vi "Parse Full Path or Item Name.vi"(11 "Full Path (with $) or Name":string) -> (3 "Relative Path or JSON-format name":string)   [LabVIEW 2017, in "JSONtext.lvlib"]
uses:
  JSONtext.lvlib
  support/quote and escape json string 2.vi
  <vilib>/JDP Science/JDP Science Common Utilities/JDP Utility.lvlib
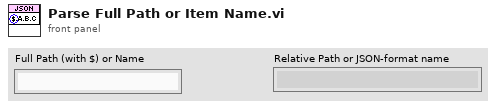
[diagram p1: front panel]
types:
  T1 = typedef "JSONtext.lvlib/Parsing State.ctl" = enum16{"Parser Error", "Object", "Array", "String", "Number/Other", "Leading Whitespace", "Object end", "Array end", "Value end"}
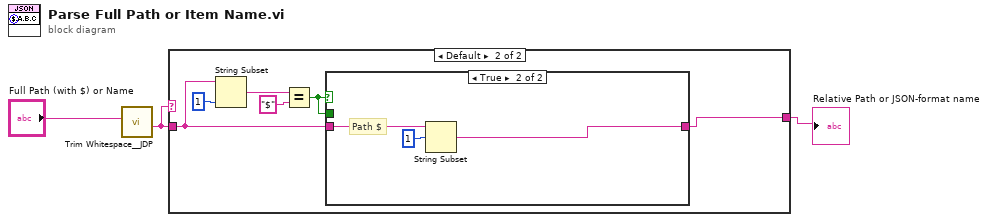
[diagram p0: block diagram]
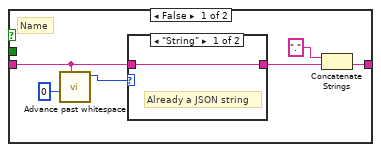
[diagram p3: hidden frame]
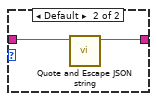
[diagram p4: hidden frame]
diagram:
  n1 = call <vilib>:"Trim Whitespace__JDP.vi"("String in"="Full Path (with $) or Name") -> ("String out"=w2:string)  [unwired: 6 in]
  n2 = case shown="Default" w2 {
    tunnel: w2 -> [_ w5]
    tunnel: [_ w4] -> w1
    frame "" {
    }
    frame Default {
      n3 = String Subset(string=w5, length (rest)=1 ("length (rest)")) -> (substring=w9:string)  [unwired: 1 in]
      n4 = Equal?(x=w9, y="$") -> (x = y?=w6:bool)
      n5 = case shown="True" w6 {
        tunnel: w6 -> [_ _]
        tunnel: w5 -> [w15 w21]
        tunnel: [w10 w19] -> w4
        frame False {
          # "Name"
          n6 = call "Advance past whitespace.vi"("JSON"=w15, "Offset"=0) -> ("Parser State"=w13:T1)  [unwired: 8 in, 1 out]
          n7 = case shown="\"String\"" w13 {
            tunnel: [w16 w18] -> w11
            tunnel: w15 -> [w16 w17]
            frame "String" {
              # "Already a JSON string"
            }
            frame Default {
              n8 = call "Quote and Escape JSON string.vi"("Plain Text"=w17) -> ("<JSON>"=w18:string)  [unwired: 10 in]
            }
          }
          n9 = Concatenate Strings("." ("string"), w11) -> (w10:string)
        }
        frame True {
          # "Path $"
          n10 = String Subset(string=w21, offset (0)=1) -> (substring=w19:string)  [unwired: 1 in]
        }
      }
    }
  }
  "Relative Path or JSON-format name" <- w1
